vi "test_generic.vi"() -> ()   [LabVIEW 2010, in "GenericSegmenter.lvclass"]
uses:
  GenericSegmenter.lvclass
  common/classes/ImageCollection/ImageCollection/ImageCollection.lvclass
  common/classes/GenericComponent/GenericComponent/GenericComponent.lvclass
  common/classes/Image/Image/Image.lvclass
  common/classes/ImageCollection/ImageCollection/add_mode_enum.ctl
panel:
  in  "frame":i32(slide) scale=1.0..1.1
  in  "loadButton":bool
  out "original image":T1(plugin-control)
  in  "segmentButton":bool
  in  "stopButton":bool
  in  "createButton":bool
  # "Test for Segmenter Classes"
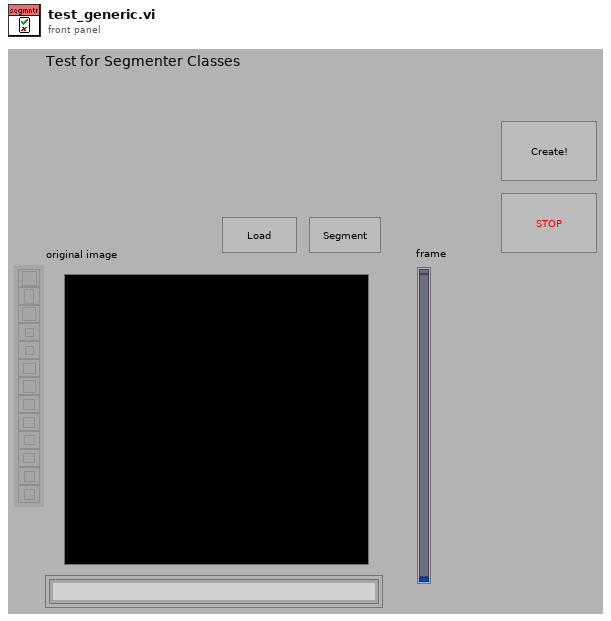
[diagram p1: front panel]
types:
  T1 = typedef "IMAQ Image.ctl" = refnum<image>
  T2 = typedef "ImageCollection.lvclass/add_mode_enum.ctl" = enum16{"instance", "copy"}
  T3 = typedef "XComponentSpecification.xctl/data.ctl" = cluster{"class path":string, "configuration":string, "label":string, "settings name":string}
  T4 = typedef "Image Type" = u32
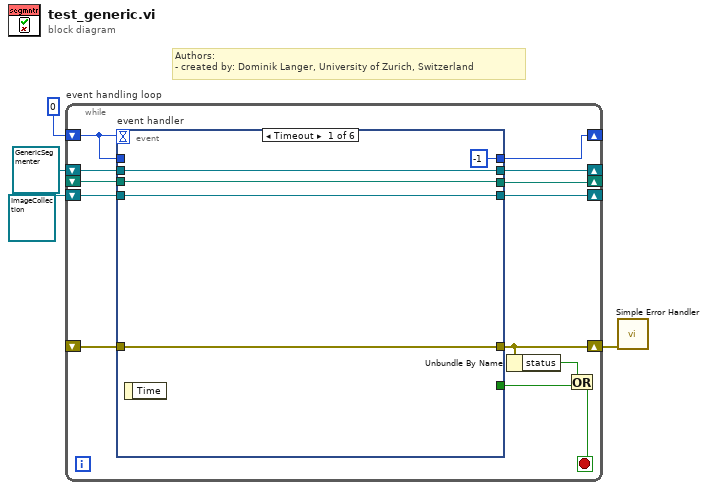
[diagram p0: block diagram]
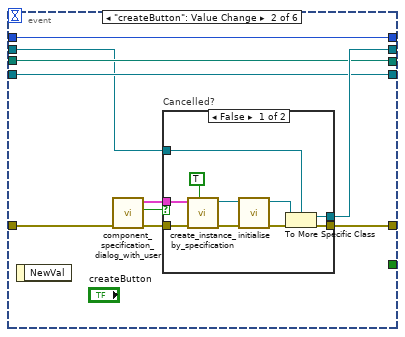
[diagram p2: hidden frame]
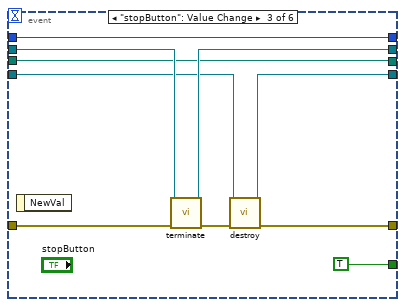
[diagram p4: hidden frame]
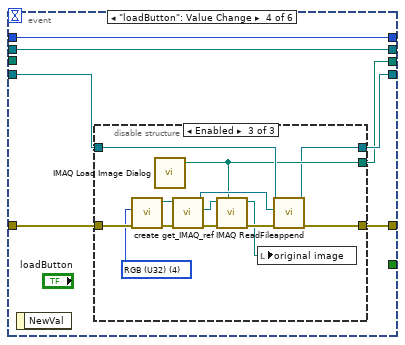
[diagram p5: hidden frame]
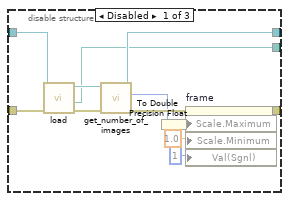
[diagram p6: hidden frame]
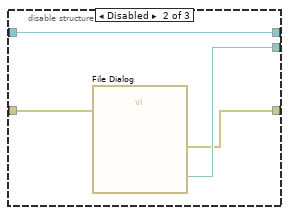
[diagram p7: hidden frame]
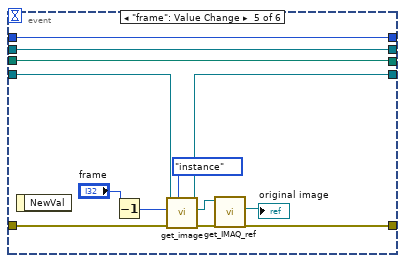
[diagram p8: hidden frame]
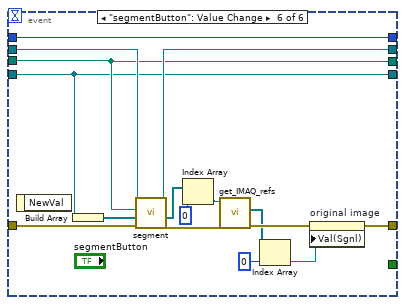
[diagram p9: hidden frame]
diagram:
  # "Authors: \n- created by: Dominik Langer, University of Zurich, Switzerland"
  n1 = while "event handling loop" {
    shift-right: [w16] -> w4
    shift-left: _ -> [w17]
    shift-right: [w12] -> _
    shift-left: refnum<class "GenericSegmenter.lvclass"> refnum ("GenericPlugin out") -> [w11]
    shift-right: [w9] -> _
    shift-left: refnum<class "ImageCollection.lvclass"> refnum ("ImageCollection.lvclass") -> [w10]
    shift-right: [w8] -> _
    shift-left: _ -> [w7]
    shift-right: [w5] -> _
    shift-left: 0 -> [w6]
    stop <- w13 stop-if-true
    n2 = event "event handler" shown="[0] Timeout" {
      selector: _ -> [_ _ _ _ _ _]
      dyn-events: _ -> [_ _ _ _ _ _]
      timeout: w6 -> [_ _ _ _ _ _]
      tunnel: w17 -> [w18 w27 w53 w57 w100 w118]
      tunnel: [w18 w32 w49 w58 w95 w112] -> w16
      tunnel: [_ _ TRUE _ _ _] -> w14
      tunnel: [w21 w31 w51 w61 w103 w119] -> w12
      tunnel: w11 -> [w21 w24 w52 w61 w103 w117]
      tunnel: [w22 w30 w47 w59 w97 w113] -> w9
      tunnel: w10 -> [w22 w30 w48 w60 w98 w113]
      tunnel: [w20 w29 w46 w56 w92 w116] -> w8
      tunnel: w7 -> [w20 w29 w46 _ w92 w116]
      tunnel: [-1 w28 w45 w55 w91 w115] -> w5
      tunnel: w6 -> [_ w28 w45 w55 w91 w115]
      event Timeout {
        n3 = event-data() -> ()  [unwired: 1 in, 1 out]
      }
      event "createButton": Value Change {
        n4 = event-data() -> ()  [unwired: 1 in, 1 out]
        n5 = call "component_specification_dialog_with_user.vi"("error in (no error)"=w27) -> ("error out"=w26:errorcluster, "cancelled?"=w23:bool, "component specification out"=w25:T3)  [unwired: 8 in]
        n6 = case "Cancelled?" shown="False" w23 {
          tunnel: [w38 w43] -> w32
          tunnel: [w36 w44] -> w31
          tunnel: w26 -> [w35 w43]
          tunnel: w25 -> [w34 _]
          tunnel: w24 -> [w33 w44]
          frame False {
            n7 = call "create_instance_by_specification.vi"("call constructor?"=TRUE, "error in (no error)"=w35, "component specification"=w34) -> ("error out"=w41:errorcluster, "GenericPlugin out"=w40:refnum<class "GenericComponent.lvclass">)  [unwired: 6 in, 1 out]
            n8 = call-dynamic "initialise.vi"("error in (no error)"=w41, "GenericPlugin in"=w40) -> ("error out"=w39:errorcluster, "GenericPlugin out"=w37:refnum<class "GenericComponent.lvclass">)  [unwired: 8 in]
            n9 = To More Specific Class(target class=w33, reference=w37, error in=w39) -> (specific class reference=w36:refnum<class "GenericSegmenter.lvclass">, error out=w38:errorcluster)
          }
          frame True {
          }
        }
      }
      event "stopButton": Value Change {
        n10 = event-data() -> ()  [unwired: 1 in, 1 out]
        n11 = call-dynamic "terminate.vi"("error in (no error)"=w53, "GenericPlugin in"=w52) -> ("error out"=w50:errorcluster, "GenericPlugin out"=w51:refnum<class "GenericSegmenter.lvclass">)  [unwired: 8 in]
        n12 = call-dynamic "destroy.vi"("error in (no error)"=w50, "ImageCollection in"=w48) -> ("error out"=w49:errorcluster, "ImageCollection out"=w47:refnum<class "ImageCollection.lvclass">)  [unwired: 8 in]
      }
      event "loadButton": Value Change {
        n13 = event-data() -> ()  [unwired: 1 in, 1 out]
        n14 = disable-structure shown="Enabled" {
          disable-tunnel: w60 -> [w73 w74 w83]
          disable-tunnel: [w70 w74 w79] -> w59
          disable-tunnel: [w68 w75 w80] -> w58
          disable-tunnel: w57 -> [w63 w77 w90]
          disable-tunnel: [w62 w76 w81] -> w56
          frame Disabled {
            n15 = call "load.vi"("error in (no error)"=w63, "ImageCollection in"=w73) -> ("error out"=w72:errorcluster, "path out"=w62:path, "ImageCollection out"=w71:refnum<class "ImageCollection.lvclass">)  [unwired: 5 in, 2 out]
            n16 = call-dynamic "get_number_of_images.vi"("error in (no error)"=w72, "ImageCollection in"=w71) -> ("error out"=w69:errorcluster, "size"=w67:i32, "ImageCollection out"=w70:refnum<class "ImageCollection.lvclass">)  [unwired: 7 in]
            n17 = To Double Precision Float(number=w67) -> (double precision float=w66:dbl)
            n18 = property on="frame" class="Slide (strict)"(error in=w69, "Scale.Maximum"=w66, "Scale.Minimum"=1.0 ("Scale.Range:Minimum"), "Val(Sgnl)"=1 ("Value (Signaling)")) -> (error out=w68:errorcluster)  [unwired: 1 in, 1 out]
          }
          frame Disabled {
            n19 = call "File Dialog"("error in"=w77) -> ("selected path"=w76:path, "error out"=w75:errorcluster)  [unwired: 11 in, 2 out]
          }
          frame Enabled {
            w89 = T4 4 items=["Grayscale (U8)", "Grayscale (I16)", "Grayscale (SGL)", "Complex (CSG)", "RGB (U32)", "HSL (U32)", "RGB (U64)", "Grayscale (U16)"] ("Image Type")
            n20 = call "create.vi"("error in (no error)"=w90, "Image Type"=w89) -> ("error out"=w88:errorcluster, "Image out"=w86:refnum<class "Image.lvclass">)  [unwired: 8 in]
            n21 = call "IMAQ Load Image Dialog"() -> ("Path"=w81:path)  [unwired: 9 in, 2 out]
            n22 = call-dynamic "get_IMAQ_ref.vi"("error in (no error)"=w88, "Image.lvclass in"=w86) -> ("error out"=w87:errorcluster, "Image"=w85:T1, "Image.lvclass out"=w82:refnum<class "Image.lvclass">)  [unwired: 5 in, 2 out]
            n23 = call "IMAQ ReadFile"("File Path"=w81, "error in (no error)"=w87, "Image"=w85) -> ("error out"=w84:errorcluster, "Image Out"=w78:T1)  [unwired: 4 in, 3 out]
            n24 = local write "original image"(w78) -> ()
            n25 = call-dynamic "append.vi"("error in (no error)"=w84, "Image.lvclass"=w82, "ImageCollection in"=w83) -> ("error out"=w80:errorcluster, "ImageCollection out"=w79:refnum<class "ImageCollection.lvclass">)  [unwired: 6 in, 1 out]
          }
        }
      }
      event "frame": Value Change {
        n26 = event-data() -> ()  [unwired: 1 in, 1 out]
        n27 = Decrement(x="frame") -> (x-1=w101:i32)
        n28 = call-dynamic "get_image.vi"("get image as..."=add_mode_enum."instance", "error in (no error)"=w100, "index"=w101, "ImageCollection in"=w98) -> ("error out"=w96:errorcluster, "Image.lvclass"=w94:refnum<class "Image.lvclass">, "ImageCollection out"=w97:refnum<class "ImageCollection.lvclass">)  [unwired: 5 in]
        n29 = call-dynamic "get_IMAQ_ref.vi"("error in (no error)"=w96, "Image.lvclass in"=w94) -> ("error out"=w95:errorcluster, "Image"=→"original image":T1)  [unwired: 5 in, 3 out]
      }
      event "segmentButton": Value Change {
        n30 = event-data() -> ()  [unwired: 1 in, 1 out]
        n31 = Build Array(w113) -> (w114:refnum<class "ImageCollection.lvclass">[])
        n32 = call-dynamic "segment.vi"("error in (no error)"=w118, "ImageCollection in"=w114, "image file path"=w116, "GenericSegmenter in"=w117) -> ("error out"=w111:errorcluster, "ImageCollection out"=w109:refnum<class "ImageCollection.lvclass">[], "GenericSegmenter out"=w119:refnum<class "GenericSegmenter.lvclass">)  [unwired: 3 in, 2 out]
        n33 = Index Array(array=w109, index=0) -> (element=w108:refnum<class "ImageCollection.lvclass">)
        n34 = call-dynamic "get_IMAQ_refs.vi"("error in (no error)"=w111, "ImageCollection in"=w108) -> ("error out"=w110:errorcluster, "IMAQ refs"=w106:T1[])  [unwired: 7 in, 1 out]
        n35 = Index Array(array=w106, index=0) -> (element=w105:T1)
        n36 = property on="original image" class="ImageControl"(error in=w110, "Val(Sgnl)"=w105) -> (error out=w112:errorcluster)  [unwired: 1 in, 1 out]
      }
    }
    n37 = Unbundle By Name(w16) -> ("status"=w15:bool)
    n38 = Or(x=w15, y=w14) -> (x .or. y?=w13:bool)
  }
  n39 = call <vilib>:"Simple Error Handler.vi"("error in (no error)"=w4) -> ()  [unwired: 4 in, 5 out]
